vi "Get Behavior Flags.vi"(8 "error in (no error)":errorcluster, 11 "Data Item in":refnum<class "Data Item.lvclass">) -> (0 "error out":errorcluster, 2 "Behavior":T1={"Children"=enum."None", "Editable"=TRUE, "XML uses />"=FALSE}, 3 "Data Item out":refnum<class "Data Item.lvclass">)   [LabVIEW 2023, in "VILab.lvlib" / "Data Item.lvclass"]
uses:
  Data Item.lvclass
  Behavior Flags.ctl
  Child Support.ctl
  Data Item.lvclass/Data Item.ctl
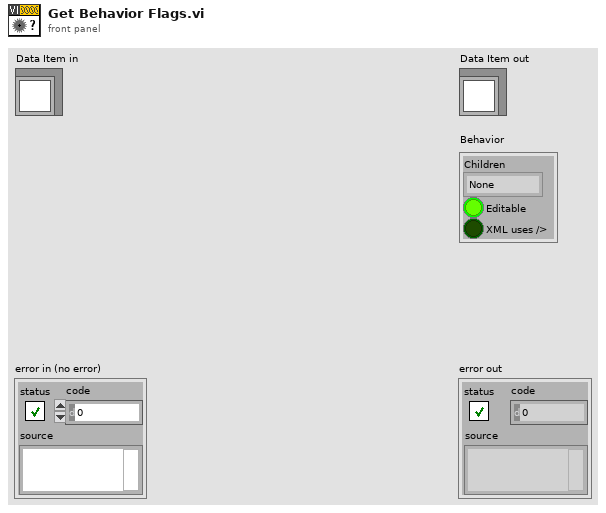
[diagram p1: front panel]
types:
  T1 = typedef "VILab.lvlib/Data Item.lvclass/Behavior Flags.ctl" = cluster{"Children":T2, "Editable":bool, "XML uses />":bool}
  T2 = typedef "VILab.lvlib/Data Item.lvclass/Child Support.ctl" = enum16{"None", "One", "At most one", "Multiple"}
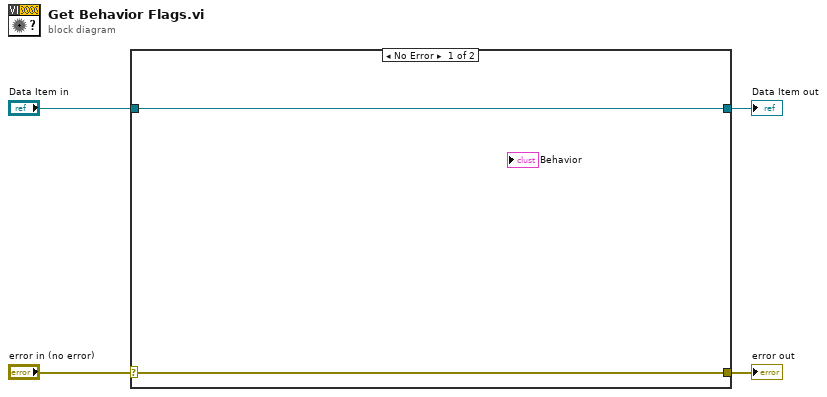
[diagram p0: block diagram]
diagram:
  n1 = case shown="No Error" "error in (no error)" {
    selector: "error in (no error)" -> [w5 w8]
    tunnel: [w5 w8] -> w3
    tunnel: [w6 w7] -> w1
    tunnel: "Data Item in" -> [w6 w7]
    frame No Error {
    }
    frame Error {
    }
  }
  "error out" <- w3
  "Data Item out" <- w1
